vi "Save Load Instrument Settings.vi"(7 "Operation (0: Save)":u16(ring) items=["Save", "Load"], 8 "error in (no error)":errorcluster, 10 "Setting File Name (Setting0.TFS)":string="Setting0.TFS", 11 "VISA resource name":refnum<visa-resource-name>) -> (0 "error out":errorcluster, 3 "VISA resource name out":refnum<visa-resource-name>)   [LabVIEW 2013, in "AWG.lvlib" / "Tektronix AFG 3000 Series.lvlib"]
doc: "Saves the current setting (last setup memory, setup memory 0) to the file in the usb memory or copies a setup file in the usb storage to an internal setup\nMemory 0 (last setup memory), and recall it.\n\nNote:\nThis VI is only applicable for AFG 3KC Series.\nAFG3252C, AFG3251C, AFG3102C, AFG3101C, AFG3052C, AFG3051C, AFG3022C, AFG3021C, AFG3011C."
uses:
  Tektronix AFG 3000 Series.lvlib
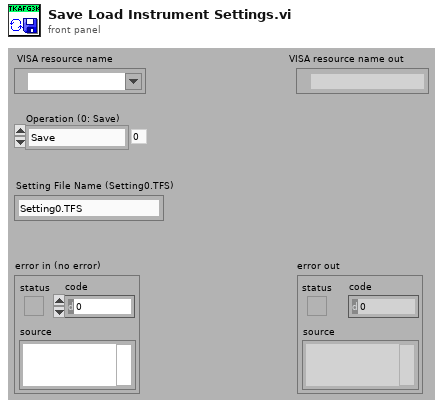
[diagram p1: front panel]
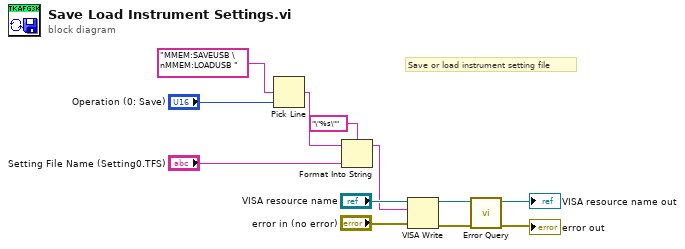
[diagram p0: block diagram]
diagram:
  # "Save or load instrument setting file"
  n1 = Pick Line(multi-line string="MMEM:SAVEUSB \nMMEM:LOADUSB " ("string (\"\")"), line index="Operation (0: Save)") -> (output string=w8:string)  [unwired: 1 in]
  n2 = Format Into String(format string="\"%s\"" ("string (\"\")"), initial string=w8, "Setting File Name (Setting0.TFS)") -> (resulting string=w3:string)  [unwired: 1 in, 1 out]
  n3 = VISA Write(VISA resource name="VISA resource name", write buffer=w3, error in (no error)="error in (no error)") -> (VISA resource name out=w7:refnum<visa-resource-name>, error out=w6:errorcluster)  [unwired: 1 out]
  n4 = call "Error Query.vi"("error in (no error)"=w6, "VISA resource name"=w7) -> ("error out"=→"error out":errorcluster, "VISA resource name out"=→"VISA resource name out":refnum<visa-resource-name>)  [unwired: 6 in, 2 out]
